vi "MAJ_Graphe.vi"(0 "Horodatage":timestamp[](array[timestamp]), 1 "Donnees":dbl[][](array[numeric]), 3 "Entetes colonnes":string[](array[string])) -> (6 "Graphe":T1(graph), 9 "Paramètres à afficher":string[](array[string]))   [LabVIEW 2013]
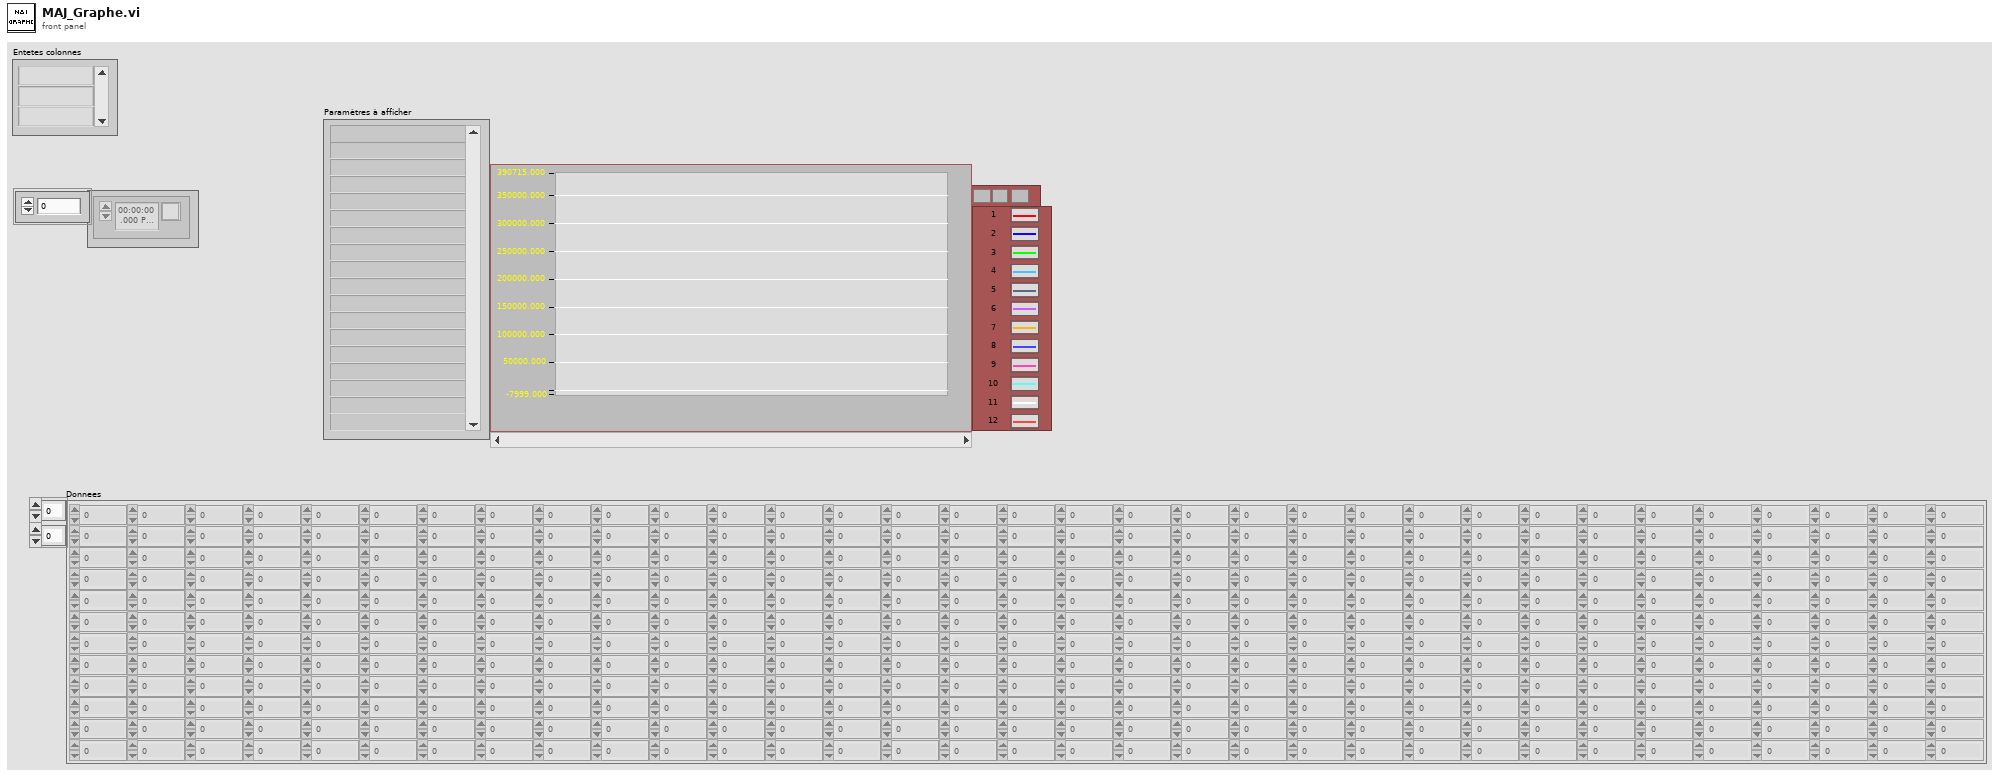
[diagram p1: front panel]
types:
  T1 = cluster{"Horodatage":timestamp[], "Donnees":dbl[]}[]
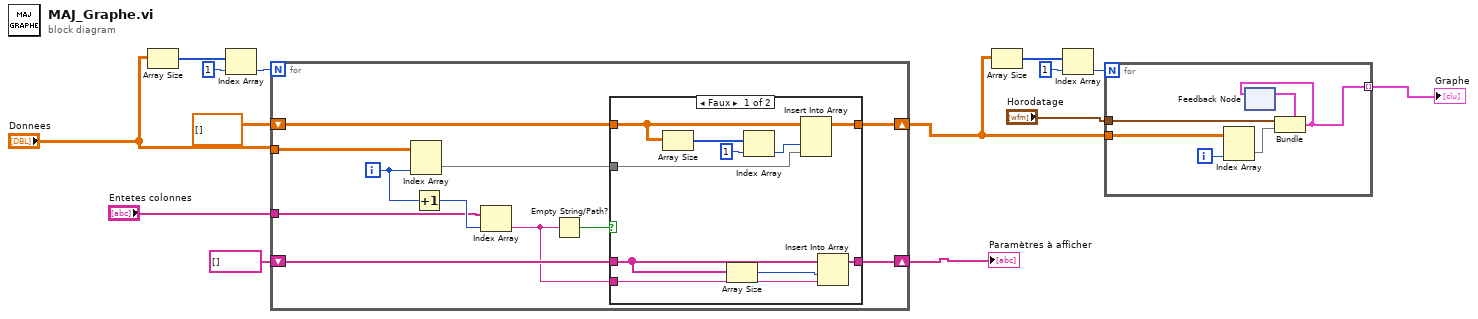
[diagram p0: block diagram]
diagram:
  n1 = Array Size(array="Donnees") -> (size(s)=w10:i32[])
  n2 = Index Array(array=w10, index=1 ("indice")) -> (element=w9:i32)
  n3 = for {
    N: w9 -> [_]
    tunnel: "Donnees" -> [w25]
    shift-right: [w19] -> w7
    shift-left: dbl[][] [] -> [w20]
    shift-right: [w18] -> w5
    shift-left: string[] [] -> [w17]
    tunnel: "Entetes colonnes" -> [w16]
    i -> [w22]
    n4 = Index Array(array=w25, index (col)=w22) -> (element=w21:dbl[])  [unwired: 1 in]
    n5 = Increment(x=w22) -> (x+1=w24:i32)
    n6 = Index Array(array=w16, index=w24) -> (element=w15:string)
    n7 = Empty String/Path?(string/path=w15) -> (empty?=w23:bool)
    n8 = case shown="Faux" w23 {
      tunnel: w21 -> [w35 _]
      tunnel: w20 -> [w31 w37]
      tunnel: [w34 w37] -> w19
      tunnel: w17 -> [w28 w36]
      tunnel: [w29 w36] -> w18
      tunnel: w15 -> [w26 _]
      frame False {
        n9 = Array Size(array=w31) -> (size(s)=w33:i32[])
        n10 = Array Size(array=w28) -> (size(s)=w27:i32)
        n11 = Index Array(array=w33, index=1 ("indice")) -> (element=w30:i32)
        n12 = Insert Into Array(array=w31, index (col)=w30, new element=w35) -> (w34:dbl[][])  [unwired: 1 in]
        n13 = Insert Into Array(array=w28, index=w27, new element=w26) -> (w29:string[])
      }
      frame True {
      }
    }
  }
  "Paramètres à afficher" <- w5
  n14 = Array Size(array=w7) -> (size(s)=w14:i32[])
  n15 = Index Array(array=w14, index=1 ("indice")) -> (element=w13:i32)
  n16 = for {
    N: w13 -> [_]
    tunnel: "Horodatage" -> [w43]
    tunnel: w7 -> [w42]
    tunnel: [w38] -> w4 mode=indexing
    i -> [w39]
    n17 = Index Array(array=w42, index (col)=w39) -> (element=w40:dbl[])  [unwired: 1 in]
    n18 = feedback #1() -> (w41:cluster{"Horodatage":timestamp[], dbl[]})  [unwired: 1 in]
    n19 = Bundle(cluster=w41, "Horodatage"=w43, w40) -> (w38:cluster{"Horodatage":timestamp[], dbl[]})
    n20 = feedback-in #1(w38) -> ()
  }
  "Graphe" <- w4
